vi "Constants.vi"() -> ()   [LabVIEW 2015]
panel:
  out "anglePID":T1
  in  "Aim Angle Offset":dbl
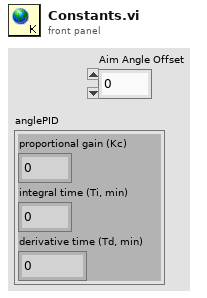
[diagram p1: front panel]
types:
  T1 = cluster{"proportional gain (Kc)":dbl, "integral time (Ti, min)":dbl, "derivative time (Td, min)":dbl}
diagram:
